vi "Get Physical Units from TD.vi"(8 "错误输入":errorcluster, 10 "float or Array Type Desciptor":T2) -> (0 "错误输出":errorcluster, 2 "Physical Units":T1[](array[typedef]))   [LabVIEW 2012, in "TD Tools.lvlib"]
uses:
  TD Tools.lvlib
  Custom Type/Type Descriptor.ctl
  Custom Type/Physical Units.ctl
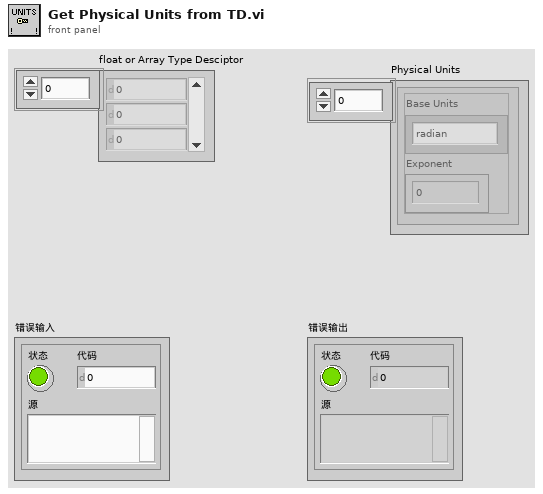
[diagram p1: front panel]
types:
  T1 = typedef "TD Tools.lvlib/Physical Units.ctl" = cluster{"Base Units":enum16{"radian", "steradian", "second", "meter", "kilogram", "ampere", "kelvin", "mole", "candela"}, "Exponent":dbl}
  T2 = typedef "TD Tools.lvlib/Type Descriptor.ctl" = u16[]
  T3 = typedef "TD Tools.lvlib/Type Descriptor Enumeration.ctl" = enum16{"<Null>", "I8", "I16", "I32", "I64", "U8", "U16", "U32", "U64", "SGL", "DBL", "EXT", "CSG", "CDB", "CXT", "0x0F", "0x10", "0x11", "0x12", "0x13", "0x14", "Enum U8", "Enum U16", "Enum U32", "Enum U64", "SGL PQ", "DBL PQ", "EXT PQ", "CSG PQ", "CDB PQ", "CXT PQ", "0x1F", "0x20", "Boolean", "0x22", "0x23", "0x24", "0x25", "0x26", "0x27", "0x28", "0x29", "0x2A", "0x2B", "0x2C", "0x2D", "0x2E", "0x2F", "String", "0x31", "Path", "Pict", "0x34", "0x35", "0x36", "DAQ", "0x38", "0x39", "0x3A", "0x3B", "0x3C", "0x3D", "0x3E", "0x3F", "Array", "0x41", "0x42", "0x43", "0x44", "0x45", "0x46", "0x47", "0x48", "0x49", "0x4A", "0x4B", "0x4C", "0x4D", "0x4E", "0x4F", "Cluster", "0x51", "0x52", "Variant", "Waveform", "0x55", "0x56", "0x57", "0x58", "0x59", "0x5A", "0x5B", "0x5C", "0x5D", "0x5E", "0x5F", "0x60", "0x61", "0x62", "0x63", "0x64", "0x65", "0x66", "0x67", "0x68", "0x69", "0x6A", "0x6B", "0x6C", "0x6D", "0x6E", "0x6F", "Refnum"}
  T4 = typedef "Type Descriptor__ogtk.ctl" = i16[]
  T5 = typedef "TD Tools.lvlib/Type Descriptor Header.ctl" = cluster{"length":u16, "private":u8, "type":T3, "# elements":u16}
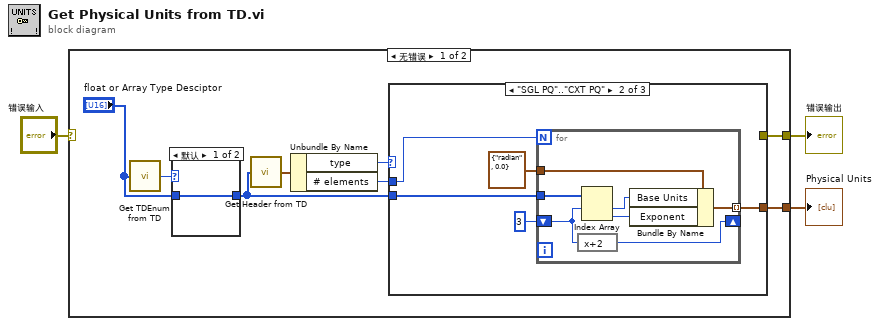
[diagram p0: block diagram]
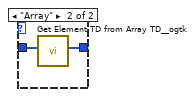
[diagram p2: hidden frame]
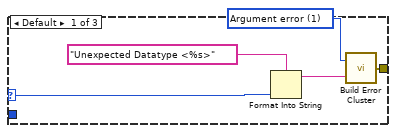
[diagram p3: hidden frame]
diagram:
  n1 = case shown="无错误" "错误输入" {
    selector: "错误输入" -> [_ w32]
    tunnel: [w11 w32] -> w2
    tunnel: [w7 _] -> w1
    frame No Error {
      n2 = call "Get TDEnum from TD.vi"("Type Descriptor"="float or Array Type Desciptor") -> ("Type Code"=w6:T3)  [unwired: 4 in]
      n3 = case shown="默认" w6 {
        tunnel: "float or Array Type Desciptor" -> [w12 w14]
        tunnel: [w12 w13] -> w5
        frame Default {
        }
        frame "Array" {
          n4 = call <userlib>:"Get Element TD from Array TD__ogtk.vi"("Array Type Descriptor"=w14) -> ("Element Type Descriptor"=w13:T4)  [unwired: 9 in, 1 out]
        }
      }
      n5 = call "Get Header from TD.vi"("Type Desciptor"=w5) -> ("Type Descriptor Header"=w10:T5)
      n6 = Unbundle By Name(w10) -> ("type"=w9:T3, "# elements"=w8:u16)
      n7 = case shown="\"SGL PQ\"..\"CXT PQ\"" w9 {
        selector: w9 -> [w16 _ _]
        tunnel: [w19 _ _] -> w11
        tunnel: w5 -> [_ w23 _]
        tunnel: w8 -> [_ w24 _]
        tunnel: [_ w21 _] -> w7
        frame Default {
          w18 = 1 items=["No error", "Argument error", "Memory is full", "Out of zone", "End of file", "File already open", "Generic file I/O error", "File not found", "File permission error", "Disk is full", "Duplicate path", "Too many files open", "System feature not enabled", "Resource file not found", "Cannot add resource", "Resource not found", "Image not found", "Image memory error", "Pen does not exist", "Config type invalid", "Config token not found", "Config parse error", "Config memory error", "Bad external code format", "Bad external code offset", "External code not present", "Null window", "Destroy window error", "Null menu", "Print aborted", "Bad print record", "Print driver error", "Windows error during printing", "Memory error during printing", "Print dialog error", "Generic print error", "Invalid device refnum", "Device not found", "Device parameter error", "Device unit error", "Cannot open device", "Device call aborted", "Generic error", "Cancelled by user", "Object ID too low", "Object ID too high", "Object not in heap", "Unknown heap", "Unknown object (invalid DefProc)", "Unknown object (DefProc not in table)", "Message out of range", "Invalid (null) method", "Unknown message", "Manager call not supported", "Bad address", "Network operation in progress", "Network operation timed out", "Connection is busy", "Network attribute not supported", "Network error", "Address in use", "System out of memory", "Connection aborted", "Connection refused", "Not connected", "Already connected", "Connection closed", "Initialization error (interapplication manager)", "Bad occurrence", "Wait on unbound occurrence handler", "Occurrence queue overflow", "Datalog type conflict", "Unused", "Unrecognized type (interapplication manager)", "Memory corrupt", "Failed to make temporary DLL", "Old CIN version", "Drag socket not found", "Failed to load drop-object", "Failed to register OLE object", "Failed to release OLE object", "Format specifier type mismatch", "Unknown format specifier", "Too few format specifiers", "Too many format specifiers", "Scan failed", "Newer CIN version", "Error converting to variant", "Runtime menu error", "Password tampered", "Variant attribute not found", "Incompatible variant data type", "Event data is not available", "Event Store is not present", "Occurrence is not found", "Event Queue is not created", "Event info is not available", "Refnum passed is NULL", "Error retrieving Class GUID", "Error retrieving CoClass GUID", "Error retrieving TypeLib GUID.", "Bad built application magic bytes.", "Specific driver is different from the specific driver associated with the Logical Name.", "There is no session opened to the class driver.", "Max Error", "MAX - Error with config objects", "MAX - Error loading configuration", "MAX - Group not supported"]
          n8 = Format Into String(format string="Unexpected Datatype <%s>" ("Format String"), w16) -> (resulting string=w15:string)  [unwired: 2 in, 1 out]
          n9 = call "Build Error Cluster.vi"("String to Prepend to source (\"\")"=w15, "code"=w18) -> ("error out"=w19:errorcluster)
        }
        frame "SGL PQ".."CXT PQ" {
          n10 = for {
            N: w24 -> [_]
            shift-right: [w26] -> _
            shift-left: 3 ("Index") -> [w27]
            tunnel: w23 -> [w31]
            tunnel: [w28] -> w21 mode=indexing
            tunnel: T1 {"Base Units"=enum."radian", "Exponent"=0.0} ("Physical Units") -> [w25]
            n11 = expression code="x+2"(w27) -> (w26:i32)
            n12 = Index Array(array=w31, index #1=w27) -> (element #1=w29:u16, element #2=w30:u16)  [unwired: 1 in]
            n13 = Bundle By Name(cluster=w25, "Base Units"=w29, "Exponent"=w30) -> (w28:T1)
          }
        }
        frame "SGL".."EXT" {
        }
      }
    }
    frame Error {
    }
  }
  "Physical Units" <- w1
  "错误输出" <- w2
